vi "Traccia_L_I.vi"() -> ()   [LabVIEW 2014]
uses:
  <vilib>/Utility/file.llb/Write To Spreadsheet File (DBL).vi
panel:
  in  "Resistenza":dbl=220.0 max=100000.0
  in  "SALVA":bool=TRUE caption="ON\nOFF"
  in  "Fondo Scala AI0":dbl(ring)=10.0 items=["10"=10.0, "5"=5.0, "0.5"=0.5, "0.05"=0.05]
  out "Segnale del fotodiodo in funzione della corrente":cluster{dbl[], dbl[]}(graph)={[0.45454545454545453, 1.0946196660482375, 1.7346938775510206, 2.374768089053803, 3.014842300556586, 3.654916512059369, 4.294990723562152, 4.9350649350649345, 5.575139146567719, 6.215213358070501, 6.855287569573285, 7.495361781076067, 8.135435992578849, 8.775510204081632, 9.415584415584414, 10.055658627087197, 10.695732838589983, 11.335807050092765, 11.975881261595546, 12.61595547309833, 13.256029684601113, 13.896103896103895, 14.536178107606679, 15.176252319109464, 15.816326530612244, 16.456400742115026, 17.09647495361781, 17.736549165120593, 18.376623376623375, 19.016697588126156, 19.656771799628938, 20.296846011131723, 20.936920222634505, 21.576994434137287, 22.217068645640076, 22.857142857142858, 23.497217068645636, 24.13729128014842, 24.777365491651203, 25.417439703153985, 26.05751391465677, 26.697588126159552, 27.337662337662334, 27.97773654916512, 28.6178107606679, 29.257884972170686, 29.897959183673468, 30.53803339517625, 31.17810760667903, 31.818181818181813], [0.00673828125, 0.00693359375, 0.006689453125, 0.0072265625, 0.0072021484375, 0.0077392578125, 0.0081298828125, 0.008251953125, 0.0092041015625, 0.0093017578125, 0.009716796875, 0.009765625, 0.0097900390625, 0.00986328125, 0.01015625, 0.0107177734375, 0.01123046875, 0.0118408203125, 0.012255859375, 0.0123291015625, 0.0125, 0.012548828125, 0.0123779296875, 0.0130126953125, 0.0130615234375, 0.0126953125, 0.0129638671875, 0.0137451171875, 0.0135009765625, 0.013720703125, 0.0144775390625, 0.0149658203125, 0.0168212890625, 0.0183349609375, 0.0189208984375, 0.0204345703125, 0.023046875, 0.0255126953125, 0.0296875, 0.0379150390625, 0.047900390625, 0.0737060546875, 0.1843017578125, 0.47919921875, 0.799072265625, 1.0858154296875, 1.331103515625, 1.5982421875, 1.9689208984375, 2.303076171875]}
  out "Vin":dbl=6.999999999999999 format="%_3g"
  out "Segnale PD":dbl=-2.303076171875 format="%_3f"
  in  "Numero misure":i16=50
  in  "Vmax":dbl=7.0 min=0.01 max=8.0 step=0.1
  in  "Vmin":dbl=0.1 min=0.01 max=8.0 step=0.1
  # "2) Collegare il CB22 all'opamp,   \n    il CB68 alla resistenza in serie al Diodo laser,\n    il CB33 alla uscita del circuito a transimpedenza del fotodiodo .\nLa terra del circuito DEVE essere in comune alla terra della scheda (CB29)."
  # "1) Selezionare il valore minimo\ned il valore massimo della tensione di \ningresso ed il numero di valori equispaziati \ntra gli estremi. Scegliere il fondo scala del CB68 e il valore della resistenza in serie al diodo laser\nPoi premere la freccetta bianca"
  # "Durante la misura gli indicatori a destra mostrano i valori di Vin e il segnale (amplificato) del fotodiodo"
  # "Sul grafico viene mostrata\nla tensione di uscita in funzione della corrente."
  # "NO\nSI"
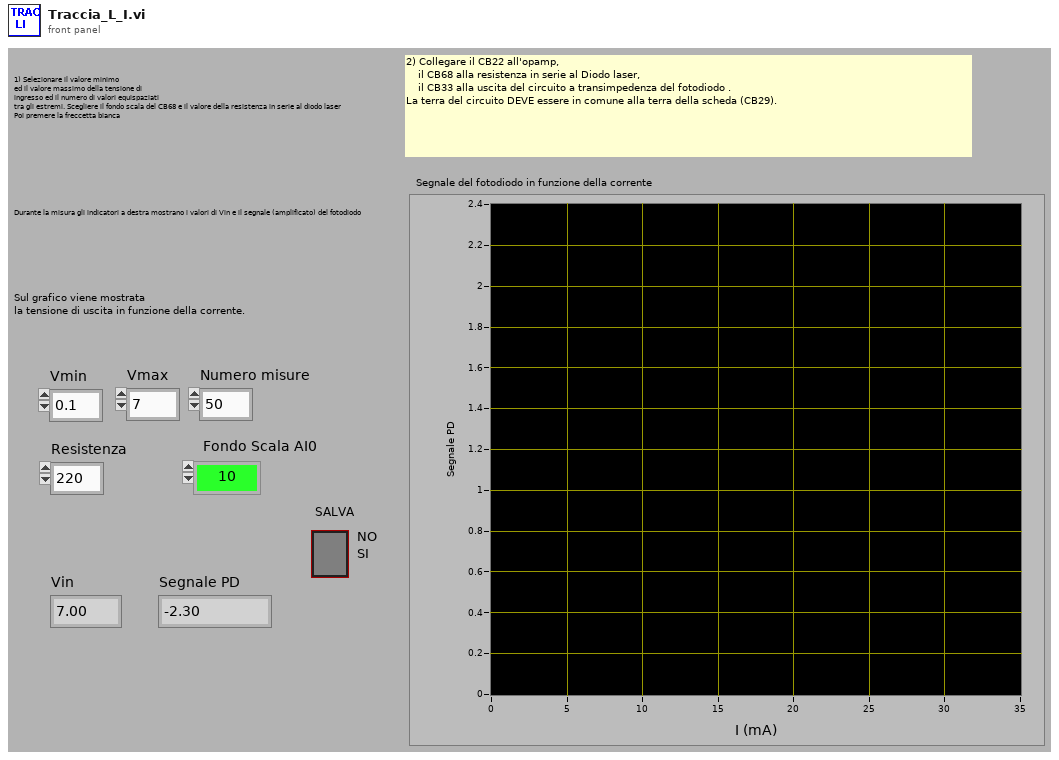
[diagram p1: front panel]
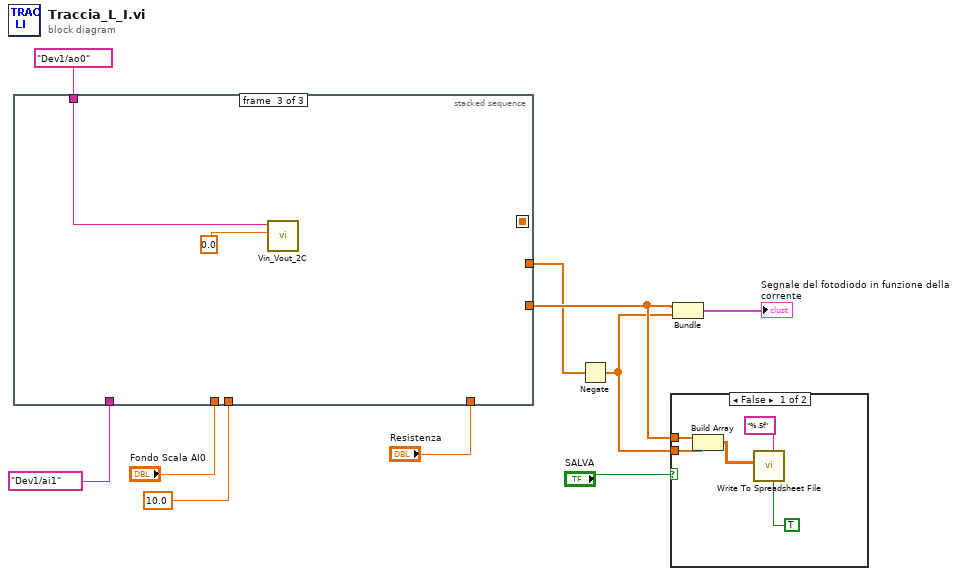
[diagram p0: block diagram]
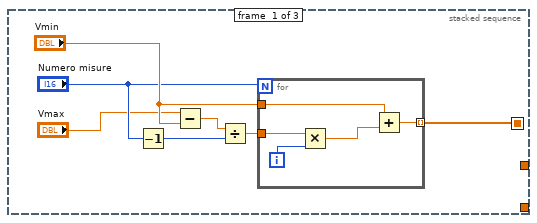
[diagram p3: hidden frame]
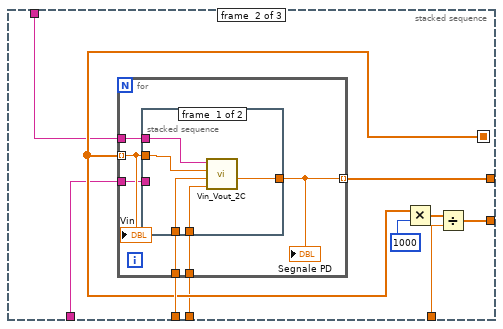
[diagram p4: hidden frame]
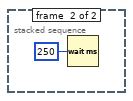
[diagram p5: hidden frame]
diagram:
  w2 = 10.0 items=["10"=10.0, "5"=5.0, "0.5"=0.5, "0.05"=0.05] ("Fondo Scala AI0 2")
  n1 = stacked-sequence {
    seq-local: [w13 _ _] -> [_ w31 _]
    tunnel: [_ w28 _] -> w9
    tunnel: "Fondo Scala AI0" -> [_ w32 _]
    tunnel: "Resistenza" -> [_ w29 _]
    tunnel: tag "Dev1/ai1" ("Canale AI") -> [_ w26 _]
    tunnel: tag "Dev1/ao0" ("Canale uscita") -> [_ w25 w46]
    tunnel: w2 -> [_ w24 _]
    tunnel: [_ w23 _] -> w1
    frame #0 {
      n2 = Decrement(x="Numero misure") -> (x-1=w16:i16)
      n3 = Subtract(x="Vmax", y="Vmin") -> (x-y=w17:dbl)
      n4 = Divide(x=w17, y=w16) -> (x/y=w15:dbl)
      n5 = for {
        N: "Numero misure" -> [_]
        tunnel: "Vmin" -> [w22]
        tunnel: [w21] -> w13 mode=indexing
        tunnel: w15 -> [w20]
        i -> [w19]
        n6 = Multiply(x=w20, y=w19) -> (x*y=w18:dbl)
        n7 = Add(x=w22, y=w18) -> (x+y=w21:dbl)
      }
    }
    frame #1 {
      n8 = for {
        tunnel: w31 -> [w38] mode=indexing
        tunnel: w32 -> [w37]
        tunnel: w26 -> [w36]
        tunnel: w25 -> [w35]
        tunnel: w24 -> [w34]
        tunnel: [w33] -> w23 mode=indexing
        n9 = stacked-sequence {
          tunnel: w38 -> [w42 _]
          tunnel: w37 -> [w41 _]
          tunnel: w36 -> [_ _]
          tunnel: w35 -> [w43 _]
          tunnel: w34 -> [w40 _]
          tunnel: [w39 _] -> w33
          frame #0 {
            n10 = call "Vin_Vout_2C.vi"("Fondo Scala AI1 (33)"=w40, "Fondo Scala AI0 (68)"=w41, "V in volt"=w42, "Canale uscita"=w43) -> ("V1 medio"=w39:dbl)  [unwired: 3 out]
          }
          frame #1 {
            n11 = Wait (ms)(milliseconds to wait=u32 250) -> ()  [unwired: 1 out]
          }
        }
        "Segnale PD" <- w33
        "Vin" <- w38
      }
      n12 = Multiply(x=w31, y=1000) -> (x*y=w30:dbl[])
      n13 = Divide(x=w30, y=w29) -> (x/y=w28:dbl[])
    }
    frame #2 {
      n14 = call "Vin_Vout_2C.vi"("V in volt"=0.0 ("V_in (Volt)"), "Canale uscita"=w46) -> ()  [unwired: 2 in, 4 out]
    }
  }
  n15 = Negate(x=w1) -> (-x=w5:dbl[])
  n16 = case shown="False" "SALVA" {
    tunnel: w5 -> [w51 _]
    tunnel: w9 -> [w50 _]
    frame False {
      n17 = Build Array(w50, w51) -> (w49:dbl[][])
      n18 = call-poly <vilib>:"Write To Spreadsheet File.vi"("transpose? (no:F)"=TRUE, "format (%.3f)"="%.5f", "2D data"=w49) -> ()  [unwired: 3 in, 3 out]
    }
    frame True {
    }
  }
  n19 = Bundle(w9, w5) -> (→"Segnale del fotodiodo in funzione della corrente":cluster{dbl[], dbl[]})  [unwired: 1 out]
